vi "Get Count and Capacity.vi"(8 "error in (no error)":errorcluster caption="错误输入（无错误）", 11 "ArrayListClass 输入":refnum<class "ArrayListClass.lvclass"> caption="DNL_LabVIEW Object in") -> (0 "error out":errorcluster caption="错误输出", 1 "Capacity":i32, 2 "Count":i32, 3 "ArrayListClass 输出":refnum<class "ArrayListClass.lvclass"> caption="DNL_LabVIEW Object out")   [LabVIEW 2012, in "ArrayListClass.lvclass"]
uses:
  ArrayListClass.lvclass
  ArrayListClass.lvclass/ArrayListClass.ctl
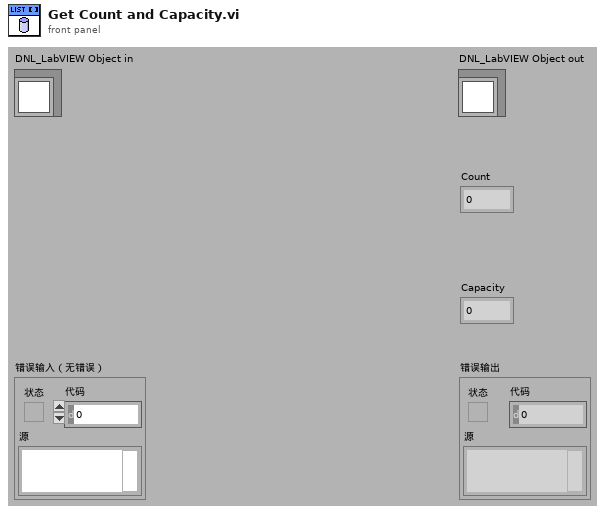
[diagram p1: front panel]
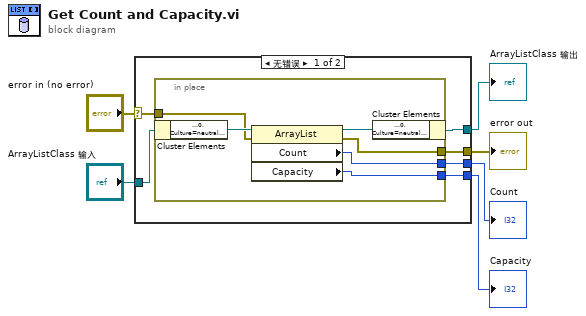
[diagram p0: block diagram]
diagram:
  n1 = case shown="无错误" "error in (no error)" {
    selector: "error in (no error)" -> [w9 w20]
    tunnel: [w8 w20] -> w5
    tunnel: [w7 w19] -> w3
    tunnel: "ArrayListClass 输入" -> [w12 w19]
    tunnel: [w11 _] -> w2
    tunnel: [w10 _] -> w1
    frame No Error {
      n2 = in-place {
        in-place-border: [w16] -> w11
        in-place-border: [w15] -> w10
        in-place-border: w9 -> [w14]
        in-place-border: [w13] -> w8
        n3 = in-place-cluster #1(w12) -> ("ArrayList"=w18:refnum<k24>)
        n4 = property class="ArrayList"(reference=w18, error in=w14) -> (reference out=w17:refnum<k24>, error out=w13:errorcluster, "Count"=w16:i32, "Capacity"=w15:i32)
        n5 = in-place-cluster #1("ArrayList"=w17) -> (w7:refnum<class "ArrayListClass.lvclass">)
      }
    }
    frame Error {
    }
  }
  "error out" <- w5
  "ArrayListClass 输出" <- w3
  "Count" <- w2
  "Capacity" <- w1
